vi "Read Test Data (DC Parallel L1N Program Mode).vi"(0 "VISA resource name":refnum<visa-resource-name>, 11 "error in (no error)":errorcluster) -> (4 "VISA resource name out":refnum<visa-resource-name>, 6 "Test Meter Data Output":T1 {"Timer" format="%.1f"; "Voltage (V)" format="%.1f"; "RMS Current (A)" format="%.3f"; "Power (W)" format="%.1f"}, 15 "error out":errorcluster)   [LabVIEW 2016, in "APT 300XAC Series.lvlib"]
doc: "Reads the DC mode <B>active data being displayed on the LCD display</B> while the test is in process. It also gives the last data taken when the test sequence compled. \n\nIn DC Mode the output data cluster has the following data.\n\n1. Memory\n2. Timer (s)\n3. Voltage (V)\n4. RMS Current (A)\n5. Power (W)\n6. Status"
uses:
  APT 300XAC Series.lvlib
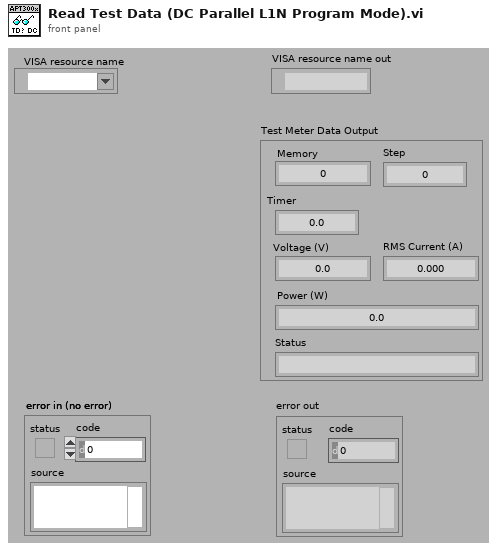
[diagram p1: front panel]
types:
  T1 = cluster{"Memory":dbl, "Voltage (V)":dbl, "RMS Current (A)":dbl, "Power (W)":dbl, "Status":string, "Timer":dbl, "Step":dbl}
  T2 = cluster{"Memory":i32, "Volt":dbl, "Current":dbl, "Power":dbl, "Status":string, "Timer":dbl, "Step":dbl}
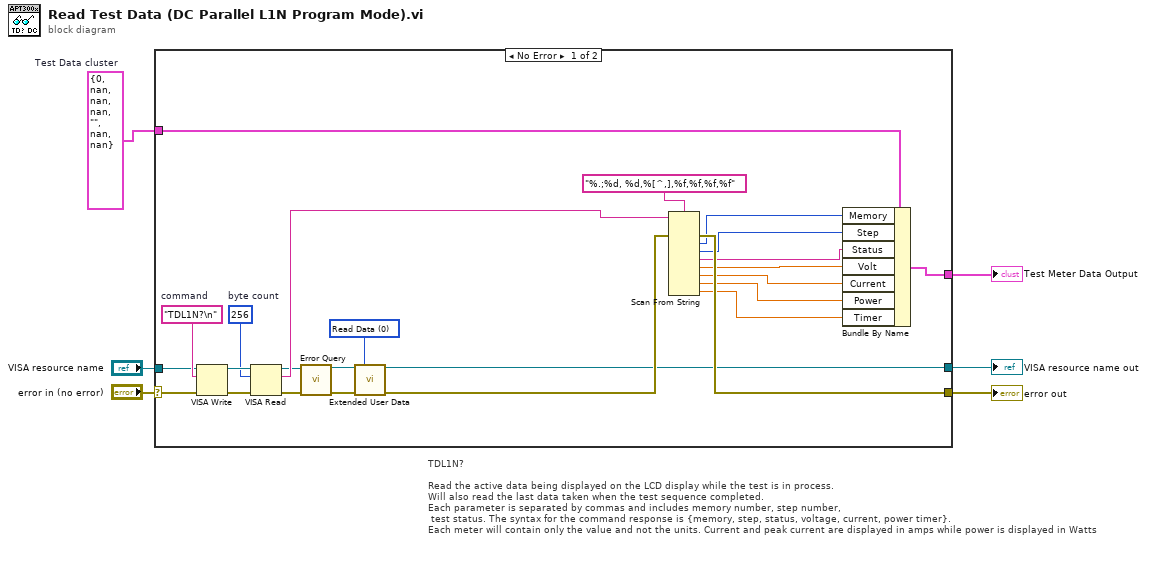
[diagram p0: block diagram]
diagram:
  w2 = T2 {"Memory"=0, "Volt"=nan, "Current"=nan, "Power"=nan, "Status"="", "Timer"=nan, "Step"=nan}  # Test Data cluster
  # "TDL1N?\n\nRead the active data being displayed on the LCD display while the test is in process. \nWill also read the last data taken when the test sequence completed. \nEach parameter is separated by commas and includes memory number, step number,\n test status. The syntax for the command response is {memory, step, status, voltage, current, power timer}. \nEach meter will contain only the value and not the units. Current and peak current are displayed in amps while power is displayed in Watts"
  n1 = case shown="No Error" "error in (no error)" {
    selector: "error in (no error)" -> [w24 w33]
    tunnel: "VISA resource name" -> [w25 w34]
    tunnel: [w15 w34] -> w4
    tunnel: [w23 w33] -> w3
    tunnel: [w28 w32] -> w1
    tunnel: w2 -> [w27 w32]
    frame No Error {
      w19 = u16 0 items=["Read Data", "Write Data", "Clear Data", "Clear ALL Data"] ("Action")
      w26 = "TDL1N?\n"  # command
      w29 = u32 256  # byte count
      n2 = VISA Write(VISA resource name=w25, write buffer=w26, error in (no error)=w24) -> (VISA resource name out=w31:refnum<visa-resource-name>, error out=w30:errorcluster)  [unwired: 1 out]
      n3 = VISA Read(VISA resource name=w31, byte count=w29, error in (no error)=w30) -> (VISA resource name out=w21:refnum<visa-resource-name>, read buffer=w22:string, error out=w20:errorcluster)  [unwired: 1 out]
      n4 = call "Error Query.vi"("VISA resource name"=w21, "error in (no error)"=w20) -> ("VISA resource name out"=w16:refnum<visa-resource-name>, "error out"=w17:errorcluster)  [unwired: 10 in, 2 out]
      n5 = call "Extended User Data.vi"("VISA resource name"=w16, "Action"=w19, "Error In (no error)"=w17) -> ("VISA resource name out"=w15:refnum<visa-resource-name>, "Error Out"=w18:errorcluster)  [unwired: 10 in, 1 out]
      n6 = Scan From String(format string="%.;%d, %d,%[^,],%f,%f,%f,%f", input string=w22, error in=w18) -> (error out=w23:errorcluster, output 1=w9:i32, output 2=w7:i32, output 3=w8:string, output 4=w13:dbl, output 5=w12:dbl, output 6=w11:dbl, output 7=w10:dbl)  [unwired: 8 in, 2 out]
      n7 = Bundle By Name(cluster=w27, "Memory"=w9, "Step"=w7, "Status"=w8, "Volt"=w13, "Current"=w12, "Power"=w11, "Timer"=w10) -> (w28:T2)
    }
    frame Error {
    }
  }
  "VISA resource name out" <- w4
  "error out" <- w3
  "Test Meter Data Output" <- w1
